vi "Connect.vi"(8 "error in (no error)":errorcluster, 11 "SolarSystems M266 Old in":refnum<class "SolarSystems M266 Old.lvclass">) -> (0 "error out":errorcluster, 3 "SolarSystems M266 Old out":refnum<class "SolarSystems M266 Old.lvclass">)   [LabVIEW 2014, in "SolarSystems M266 Old.lvclass"]
uses:
  SolarSystems M266 Old.lvclass
  SolarSystems M266 Old.lvclass/SolarSystems M266 Old.ctl
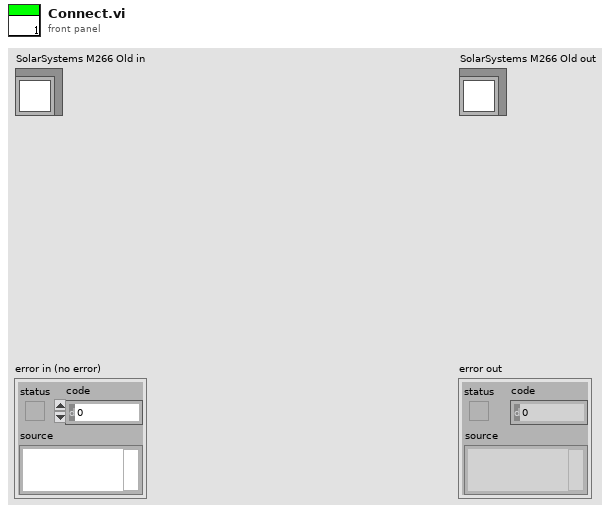
[diagram p1: front panel]
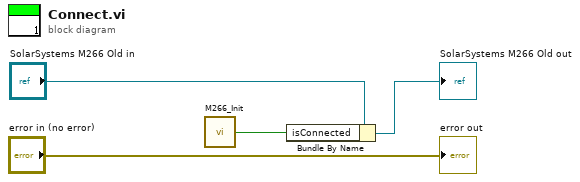
[diagram p0: block diagram]
diagram:
  n1 = call "M266_Init.vi"() -> ("Result"=w3:bool)  [unwired: 1 in]
  n2 = Bundle By Name(cluster="SolarSystems M266 Old in", "isConnected"=w3) -> (→"SolarSystems M266 Old out":refnum<class "SolarSystems M266 Old.lvclass">)
  "error out" <- "error in (no error)"
